vi "Test draw root_circle.vi"() -> ()   [LabVIEW 2020]
panel:
  in  "KML File Path":path
  out "point_hdl":i32
  out "update_count":i32
  in  "file path":path
  in  "LinePattern":refnum<k7>
  out "layer_handle":i32
  in  "CurrentZoom":i32
  in  "Lon":dbl
  in  "Lat":dbl
  out "ProjY":dbl format="%.2f"
  out "ProjX":dbl format="%#.2f"
  in  "CursorMode":i32(ring) items=["ZoomIn"=0, "cmZoomOut"=1, "Pan"=2, "cmSelection"=3, "cmNone"=4, "cmMeasure"=5, "cmAddShape"=6, "cmEditShape"=8, "cmSplitByPolyline"=9, "cmIdentify"=10, "cmMoveShapes"=11, "cmRotateShapes"=12, "cmSelectByPolygon"=13, "cmEraseByPolygon"=14, "cmSplitByPolygon"=15, "cmClipByPolygon"=16]
  out "degreesLatY":dbl
  out "degreesLngX":dbl
  in  "stop":bool
  in  "Point":refnum<k7>
  in  "Shape":refnum<k7>
  in  "Shapefile":refnum<k7>
  in  "Map":refnum<k7>(container)
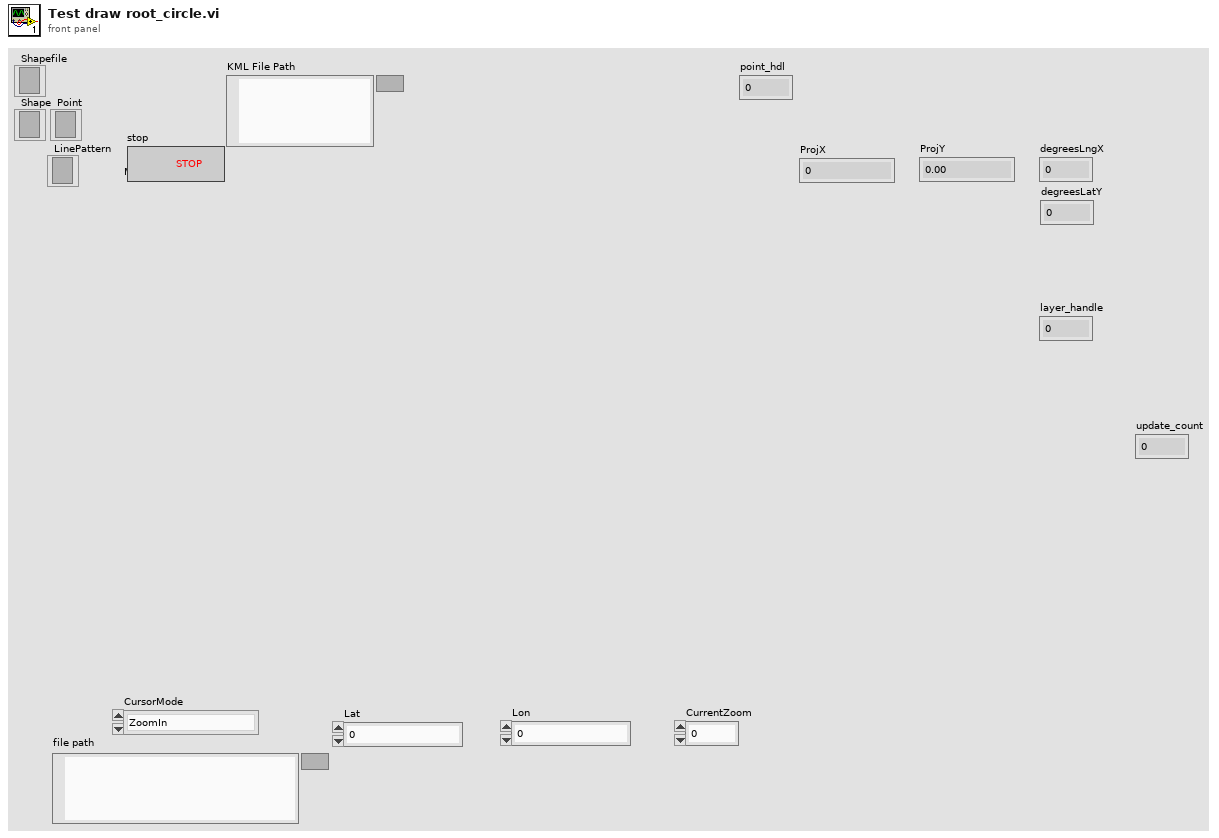
[diagram p1: front panel]
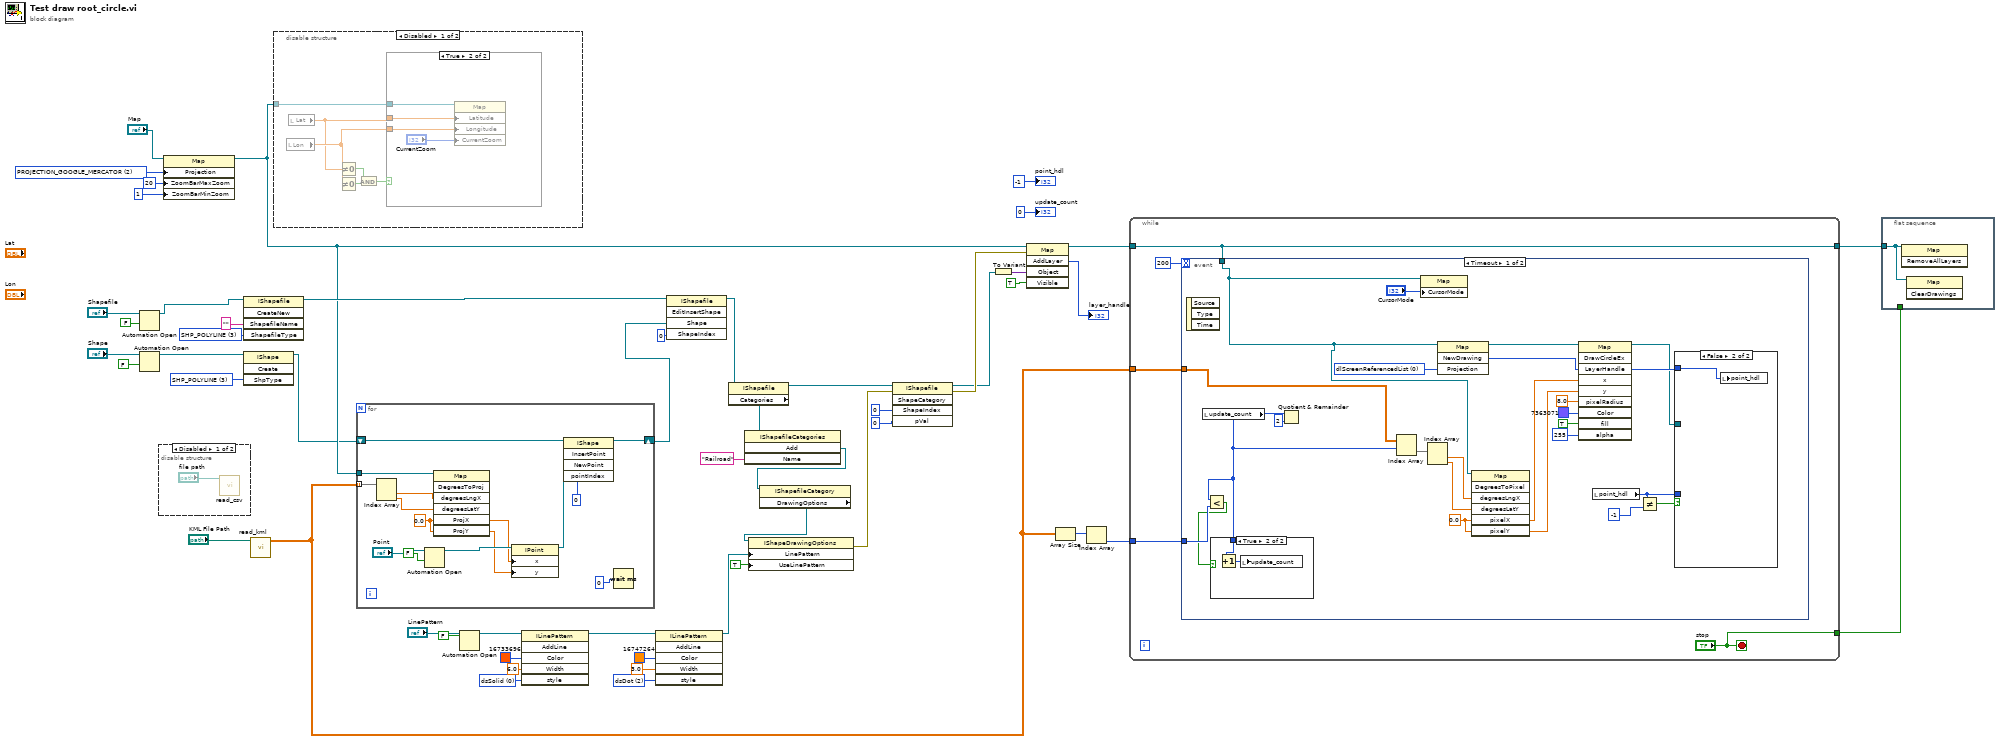
[diagram p0: block diagram]
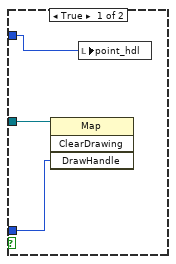
[diagram p5: hidden frame]
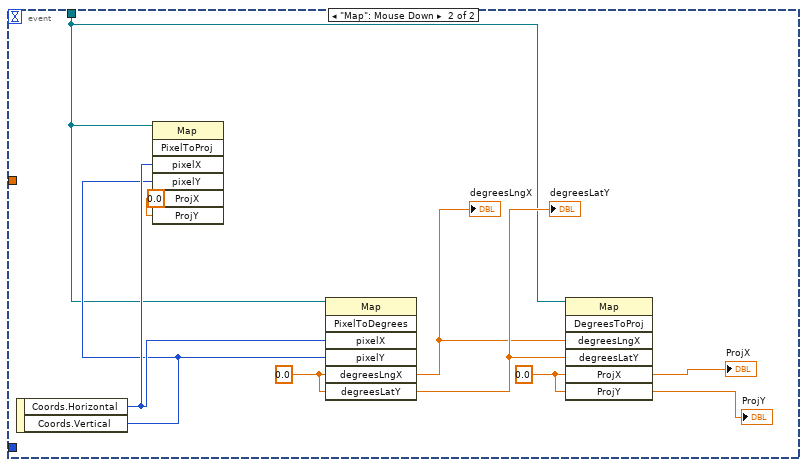
[diagram p7: hidden frame]
diagram:
  w22 = 2 items=["dsSolid", "dsDash", "dsDot", "dsDashDot", "dsDashDotDot", "dsCustom"] ("style")
  w26 = 0 items=["dsSolid", "dsDash", "dsDot", "dsDashDot", "dsDashDotDot", "dsCustom"] ("style")
  w43 = 2 items=["PROJECTION_CUSTOM"=-1, "PROJECTION_NONE"=0, "PROJECTION_WGS84"=1, "PROJECTION_GOOGLE_MERCATOR"=2] ("Projection")
  w45 = 3 items=["SHP_NULLSHAPE"=0, "SHP_POINT"=1, "SHP_POLYLINE"=3, "SHP_POLYGON"=5, "SHP_MULTIPOINT"=8, "SHP_POINTZ"=11, "SHP_POLYLINEZ"=13, "SHP_POLYGONZ"=15, "SHP_MULTIPOINTZ"=18, "SHP_POINTM"=21, "SHP_POLYLINEM"=23, "SHP_POLYGONM"=25, "SHP_MULTIPOINTM"=28, "SHP_MULTIPATCH"=31] ("ShpType")
  w47 = 3 items=["SHP_NULLSHAPE"=0, "SHP_POINT"=1, "SHP_POLYLINE"=3, "SHP_POLYGON"=5, "SHP_MULTIPOINT"=8, "SHP_POINTZ"=11, "SHP_POLYLINEZ"=13, "SHP_POLYGONZ"=15, "SHP_MULTIPOINTZ"=18, "SHP_POINTM"=21, "SHP_POLYLINEM"=23, "SHP_POLYGONM"=25, "SHP_MULTIPOINTM"=28, "SHP_MULTIPATCH"=31] ("ShapefileType")
  n1 = Automation Open(Automation Refnum="Shapefile", 9:FALSE ("open new instance (false)")) -> (Automation Refnum=w49:refnum<k7>)  [unwired: 2 in, 1 out]
  n2 = Automation Open(Automation Refnum="Shape", 9:FALSE ("open new instance (false)")) -> (Automation Refnum=w46:refnum<k7>)  [unwired: 2 in, 1 out]
  n3 = disable-structure shown="Disabled" {
    frame Disabled {
      n4 = call "read_csv.vi"("file path (dialog if empty)"="file path") -> ()  [unwired: 9 in, 2 out]
    }
    frame Enabled {
    }
  }
  n5 = property class="Map"(reference="Map", "Projection"=w43, "ZoomBarMaxZoom"=20, "ZoomBarMinZoom"=1) -> (reference out=w37:refnum<k7>)  [unwired: 1 in, 1 out]
  n6 = invoke class="IShapefile" method="CreateNew"(reference=w49, "ShapefileName"="", "ShapefileType"=w47) -> (reference out=w42:refnum<k7>)  [unwired: 2 in, 4 out]
  n7 = invoke class="IShape" method="Create"(reference=w46, "ShpType"=w45) -> (reference out=w9:refnum<k7>)  [unwired: 2 in, 3 out]
  n8 = call "read_kml.vi"("KML File Path"="KML File Path") -> ("array(lon, lat)"=w1:dbl[][])  [unwired: 9 in, 1 out]
  n9 = disable-structure shown="Disabled" {
    disable-tunnel: w37 -> [w55 _]
    frame Disabled {
      n10 = local read "Lon"() -> (w60:dbl)
      n11 = local read "Lat"() -> (w59:dbl)
      n12 = Not Equal To 0?(x=w59) -> (x != 0?=w56:bool)
      n13 = Not Equal To 0?(x=w60) -> (x != 0?=w57:bool)
      n14 = And(x=w56, y=w57) -> (x .and. y?=w58:bool)
      n15 = case shown="True" w58 {
        tunnel: w59 -> [_ w64]
        tunnel: w60 -> [_ w63]
        tunnel: w55 -> [_ w61]
        frame False {
        }
        frame True {
          n16 = property class="Map"(reference=w61, "Latitude"=w64, "Longitude"=w63, "CurrentZoom"="CurrentZoom") -> ()  [unwired: 1 in, 2 out]
        }
      }
    }
    frame Enabled {
    }
  }
  n17 = for {
    tunnel: w37 -> [w79]
    tunnel: w1 -> [w78] mode=indexing
    shift-right: [w67] -> w8
    shift-left: w9 -> [w70]
    w77 = 0.0 ("ProjX")
    n18 = Index Array(array=w78) -> (element #1=w66:dbl, element #2=w65:dbl)  [unwired: 2 in]
    n19 = Automation Open(Automation Refnum="Point", 9:FALSE ("open new instance (false)")) -> (Automation Refnum=w75:refnum<k7>)  [unwired: 2 in, 1 out]
    n20 = invoke class="Map" method="DegreesToProj"(reference=w79, "degreesLngX"=w66, "degreesLatY"=w65, "ProjX"=w77, "ProjY"=w77) -> ("ProjX"=w72:dbl, "ProjY"=w71:dbl)  [unwired: 2 in, 5 out]
    n21 = property class="IPoint"(reference=w75, "x"=w72, "y"=w71) -> (reference out=w68:refnum<k7>)  [unwired: 1 in, 1 out]
    n22 = invoke class="IShape" method="InsertPoint"(reference=w70, "NewPoint"=w68, "pointIndex"=0) -> (reference out=w67:refnum<k7>)  [unwired: 2 in, 4 out]
    n23 = Wait (ms)(milliseconds to wait=u32 0) -> ()  [unwired: 1 out]
  }
  n24 = Automation Open(Automation Refnum="LinePattern", 9:FALSE ("open new instance (false)")) -> (Automation Refnum=w29:refnum<k7>)  [unwired: 2 in, 1 out]
  n25 = invoke class="ILinePattern" method="AddLine"(reference=w29, "Color"=u32 16733696, "Width"=sgl 6.0, "style"=w26) -> (reference out=w25:refnum<k7>)  [unwired: 2 in, 5 out]
  n26 = invoke class="ILinePattern" method="AddLine"(reference=w25, "Color"=u32 16747264, "Width"=sgl 3.0, "style"=w22) -> (reference out=w21:refnum<k7>)  [unwired: 2 in, 5 out]
  n27 = invoke class="IShapefile" method="EditInsertShape"(reference=w42, "Shape"=w8, "ShapeIndex"=0) -> (reference out=w36:refnum<k7>)  [unwired: 2 in, 4 out]
  n28 = property class="IShapefile"(reference=w36) -> (reference out=w19:refnum<k7>, "Categories"=w35:refnum<k7>)  [unwired: 1 in, 1 out]
  n29 = invoke class="IShapefileCategories" method="Add"(reference=w35, "Name"="Railroad") -> ("Add"=w33:refnum<k7>)  [unwired: 2 in, 3 out]
  n30 = property class="IShapefileCategory"(reference=w33) -> ("DrawingOptions"=w32:refnum<k7>)  [unwired: 1 in, 2 out]
  n31 = property class="IShapeDrawingOptions"(reference=w32, "LinePattern"=w21, "UseLinePattern"=TRUE) -> (error out=w18:errorcluster)  [unwired: 1 in, 1 out]
  n32 = invoke class="IShapefile" method="ShapeCategory"(reference=w19, error in=w18, "ShapeIndex"=0, "pVal"=0) -> (reference out=w12:refnum<k7>, error out=w15:errorcluster)  [unwired: 1 in, 3 out]
  n33 = To Variant(anything=w12) -> (Variant=w40:variant)
  n34 = invoke class="Map" method="AddLayer"(reference=w37, error in=w15, "Object"=w40, "Visible"=TRUE) -> (reference out=w7:refnum<k7>, "AddLayer"=→"layer_handle":i32)  [unwired: 1 in, 3 out]
  n35 = Array Size(array=w1) -> (size(s)=w6:i32[])
  n36 = Index Array(array=w6) -> (element=w5:i32)  [unwired: 1 in]
  n37 = while {
    tunnel: w7 -> [w83]
    tunnel: [w83] -> w14
    tunnel: ["stop"] -> w13
    tunnel: w1 -> [w81]
    tunnel: w5 -> [w80]
    stop <- "stop" stop-if-true
    n38 = event shown="[0] Timeout" {
      selector: _ -> [_ _]
      dyn-events: _ -> [_ _]
      timeout: 200 -> [_ _]
      tunnel: w83 -> [w107 w116]
      tunnel: w81 -> [w106 _]
      tunnel: w80 -> [w105 _]
      event Timeout {
        w94 = 0.0 ("pixelX")
        w102 = 0 items=["dlScreenReferencedList", "dlSpatiallyReferencedList"] ("Projection")
        n39 = event-data() -> ()  [unwired: 1 in, 3 out]
        n40 = local read "update_count"() -> (w104:i32)
        n41 = Less?(x=w104, y=w105) -> (x < y?=w103:bool)
        n42 = case shown="True" w103 {
          tunnel: w104 -> [_ w114]
          frame False {
          }
          frame True {
            n43 = Increment(x=w114) -> (x+1=w115:i32)
            n44 = local write "update_count"(w115) -> ()
          }
        }
        n45 = Quotient & Remainder(x=w104, y=2) -> ()  [unwired: 2 out]
        n46 = Index Array(array=w106, index (row)=w104) -> (element=w95:dbl[])  [unwired: 1 in]
        n47 = property class="Map"(reference=w107, "CursorMode"="CursorMode") -> ()  [unwired: 1 in, 2 out]
        n48 = Index Array(array=w95) -> (element #1=w86:dbl, element #2=w85:dbl)  [unwired: 2 in]
        n49 = invoke class="Map" method="NewDrawing"(reference=w107, "Projection"=w102) -> (reference out=w101:refnum<k7>, "NewDrawing"=w100:i32)  [unwired: 2 in, 2 out]
        n50 = invoke class="Map" method="DegreesToPixel"(reference=w107, "degreesLngX"=w86, "degreesLatY"=w85, "pixelX"=w94, "pixelY"=w94) -> ("pixelX"=w93:dbl, "pixelY"=w92:dbl)  [unwired: 2 in, 5 out]
        n51 = invoke class="Map" method="DrawCircleEx"(reference=w101, "LayerHandle"=w100, "x"=w93, "y"=w92, "pixelRadius"=8.0, "Color"=u32 7363071, "fill"=TRUE, "alpha"=u8 255) -> (reference out=w90:refnum<k7>, "LayerHandle"=w91:i32)  [unwired: 2 in, 8 out]
        n52 = local read "point_hdl"() -> (w87:i32)
        n53 = Not Equal?(x=w87, y=-1) -> (x != y?=w88:bool)
        n54 = case shown="False" w88 {
          tunnel: w91 -> [w112 w113]
          tunnel: w90 -> [w111 _]
          tunnel: w87 -> [w110 _]
          frame True {
            n55 = invoke class="Map" method="ClearDrawing"(reference=w111, "DrawHandle"=w110) -> ()  [unwired: 2 in, 4 out]
            n56 = local write "point_hdl"(w112) -> ()
          }
          frame False {
            n57 = local write "point_hdl"(w113) -> ()
          }
        }
      }
      event "Map": Mouse Down {
        w119 = 0.0 ("ProjX")
        w124 = 0.0 ("ProjX")
        w125 = 0.0 ("degreesLngX")
        n58 = event-data() -> ("Coords.Horizontal"=w123:i32, "Coords.Vertical"=w122:i32)  [unwired: 1 in]
        n59 = invoke class="Map" method="PixelToProj"(reference=w116, "pixelX"=w123, "pixelY"=w122, "ProjX"=w124, "ProjY"=w124) -> ()  [unwired: 2 in, 7 out]
        n60 = invoke class="Map" method="PixelToDegrees"(reference=w116, "pixelX"=w123, "pixelY"=w122, "degreesLngX"=w125, "degreesLatY"=w125) -> ("degreesLngX"=w120:dbl, "degreesLatY"=w121:dbl)  [unwired: 2 in, 5 out]
        "degreesLngX" <- w120
        "degreesLatY" <- w121
        n61 = invoke class="Map" method="DegreesToProj"(reference=w116, "degreesLngX"=w120, "degreesLatY"=w121, "ProjX"=w119, "ProjY"=w119) -> ("ProjX"=→"ProjX":dbl, "ProjY"=→"ProjY":dbl)  [unwired: 2 in, 5 out]
      }
    }
  }
  n62 = flat-sequence {
    tunnel: w14 -> [w126]
    tunnel: w13 -> [_]
    frame #0 {
      n63 = invoke class="Map" method="RemoveAllLayers"(reference=w126) -> ()  [unwired: 2 in, 3 out]
      n64 = invoke class="Map" method="ClearDrawings"(reference=w126) -> ()  [unwired: 2 in, 3 out]
    }
  }
  "update_count" <- 0 ("update_count")
  "point_hdl" <- -1 ("point_hdl")
